vi "Create Connect String.vi"(11 "Channel Connection Data":T1 {"Connection Data" format="%x"}) -> (1 "Connect info string":string, 3 "Connect config string":string)   [LabVIEW 2021, in "CIFLogs.lvlib"]
uses:
  CIFLogs.lvlib
  Channels/CIFChannelMng/OOB/OOB_Rx/Typedef/Channel Connection Data.ctl
  Channels/CIFChannelMng/OOB/OOB_Rx/ChanMngOOB_Rx.lvclass
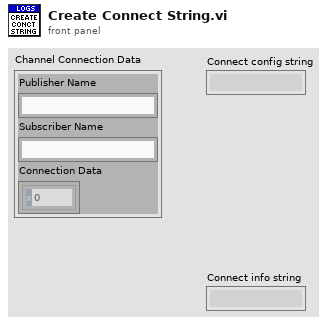
[diagram p1: front panel]
types:
  T1 = typedef "ChanMngOOB_Rx.lvclass/Channel Connection Data.ctl" = cluster{"Publisher Name":string, "Subscriber Name":string, "Connection Data":u8[]}
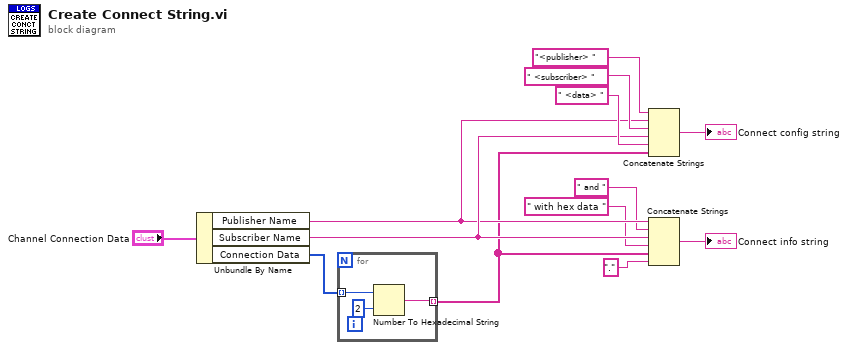
[diagram p0: block diagram]
diagram:
  n1 = Unbundle By Name("Channel Connection Data") -> ("Publisher Name"=w7:string, "Subscriber Name"=w8:string, "Connection Data"=w10:u8[])
  n2 = for {
    tunnel: w10 -> [w16] mode=indexing
    tunnel: [w14] -> w4 mode=indexing
    n3 = Number To Hexadecimal String(1:i16 2 ("width (-)"), 2:w16) -> (0:w14:string)
  }
  n4 = Concatenate Strings("<publisher> " ("string"), w7, " <subscriber> " ("string"), w8, " <data> " ("string"), w4) -> (→"Connect config string":string)
  n5 = Concatenate Strings(w7, " and " ("string"), w8, " with hex data " ("string"), w4, "." ("string")) -> (→"Connect info string":string)
